vi "create template tdms file.vi"(6 "instance name":string, 8 "error in":errorcluster, 9 "types order":T1[](array[typedef]), 10 "scans per write":i32, 11 "data dictionary in":refnum<class "data dictionary.lvclass">) -> (0 "error out":errorcluster, 2 "template path":path, 3 "data dictionary out":refnum<class "data dictionary.lvclass">)   [LabVIEW 2013, in "TDMS datalogger runtime.lvclass"]
uses:
  TDMS datalogger runtime.lvclass
  <vilib>/NI/Tag Bus/dictionary/data dictionary.lvclass
  <vilib>/NI/Tag Bus/tag/Data Type.ctl
  <vilib>/NI/LV Tools Palette/Misc/NISE Tools General.lvlib
  <vilib>/NI/Tag Bus/tag/tag descriptor.lvclass
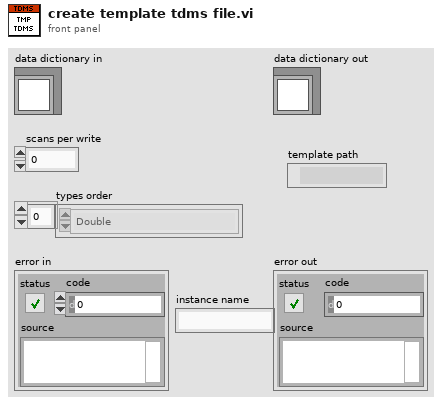
[diagram p1: front panel]
types:
  T1 = typedef "tag bus.lvlib/tag descriptor.lvclass/Data Type.ctl" = enum16{"Double", "Single", "I64", "I32", "I16", "I8", "U64", "U32", "U16", "U8", "Boolean", "String", "Array of Double", "Array of Single", "Array of I64", "Array of I32", "Array of I16", "Array of I8", "Array of U64", "Array of U32", "Array of U16", "Array of U8", "Array of Boolean", "Array of String"}
  T2 = enum16{"open", "open or create", "create or replace", "create", "open (read-only)"}
  T3 = typedef "tag bus.lvlib/data dictionary.lvclass/full data dictionary.ctl" = cluster{"Double":string[], "Single":string[], "I64":string[], "I32":string[], "I16":string[], "I8":string[], "U64":string[], "U32":string[], "U16":string[], "U8":string[], "Boolean":string[], "String":string[], "Array of Double":string[], "Array of Single":string[], "Array of I64":string[], "Array of I32":string[], "Array of I16":string[], "Array of I8":string[], "Array of U64":string[], "Array of U32":string[], "Array of U16":string[], "Array of U8":string[], "Array of Boolean":string[], "Array of String":string[]}
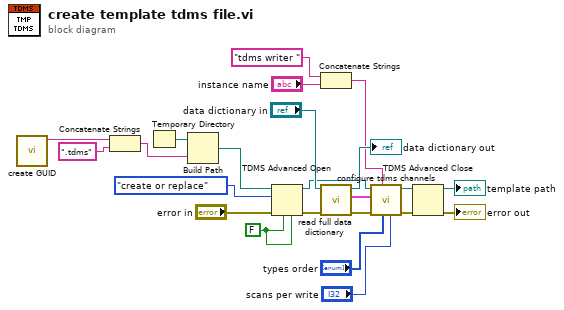
[diagram p0: block diagram]
diagram:
  w7 = FALSE ("disable buffering? (T)")
  n1 = call <vilib>:"create GUID.vi"() -> ("UUID"=w18:string)  [unwired: 11 in]
  n2 = Concatenate Strings(w18, ".tdms" ("string")) -> (w20:string)
  n3 = Temporary Directory() -> (w17:path)
  n4 = Build Path(base path=w17, name or relative path=w20) -> (appended path=w21:path)
  n5 = TDMS Advanced Open(4:w7, 6:w7, 8:"error in", 10:T2."create or replace" ("operation (0:open)"), 11:w21) -> (0:w15:errorcluster, 3:w9:refnum<k34>)  [unwired: 1 out]
  n6 = Concatenate Strings("tdms writer " ("string"), "instance name") -> (w3:string)
  n7 = call <vilib>:"read full data dictionary.vi"("error in"=w15, "data dictionary in"="data dictionary in") -> ("error out"=w11:errorcluster, "dictionary"=w10:T3, "data dictionary out"=→"data dictionary out":refnum<class "data dictionary.lvclass">)  [unwired: 7 in]
  n8 = call "configure tdms channels.vi"("samples per channel (1)"="scans per write", "type order"="types order", "group name"=w3, "error in"=w11, "dictionary"=w10, "tdms file in"=w9) -> ("error out"=w16:errorcluster, "tdms file out"=w23:refnum<k34>)  [unwired: 4 in]
  n9 = TDMS Advanced Close(8:w16, 11:w23) -> (0:→"error out":errorcluster, 3:→"template path":path)  [unwired: 2 in]
